vi "Initialize.vi"(8 "error in (no error)":errorcluster, 10 "Parameters in":refnum<class "Abstract Init Parameters.lvclass">, 11 "Abstract Consumer in":refnum<class "Abstract Consumer.lvclass">) -> (0 "error out":errorcluster, 3 "Abstract Consumer out":refnum<class "Abstract Consumer.lvclass">)   [LabVIEW 2017, in "Messaging.lvlib" / "Abstract Consumer.lvclass"]
uses:
  Abstract Consumer.lvclass
  Parameters/Abstract Init Parameters/Abstract Init Parameters.lvclass
  Abstract Consumer.lvclass/Abstract Consumer.ctl
  Message Queue/Abstract Message Queue/Abstract Message Queue.lvclass
  Messaging.lvlib
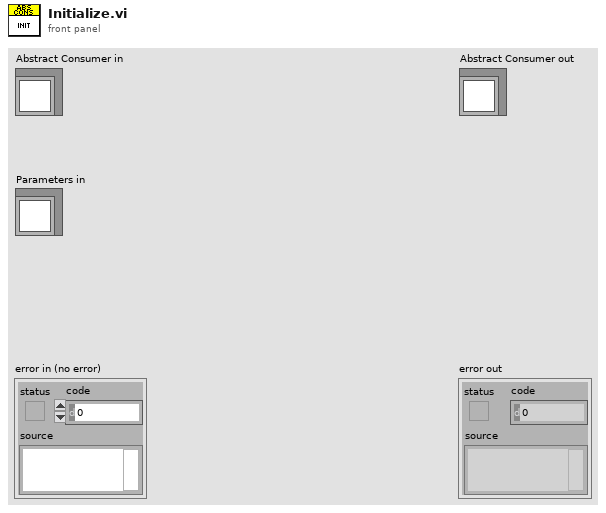
[diagram p1: front panel]
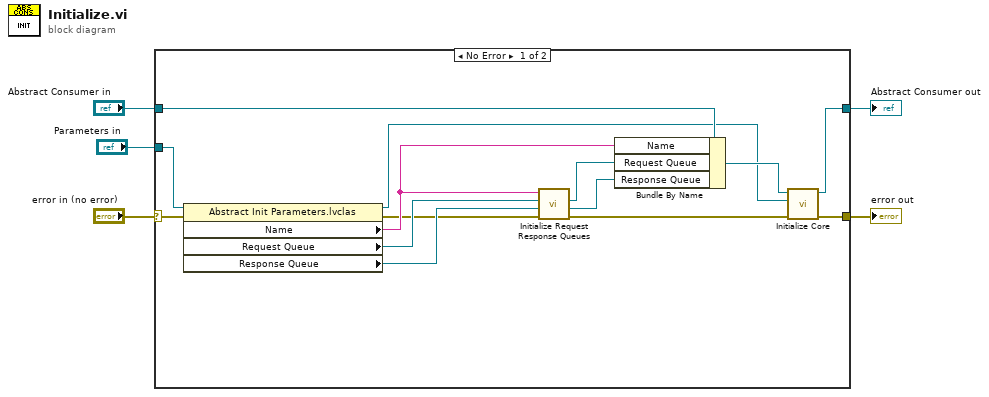
[diagram p0: block diagram]
diagram:
  n1 = case shown="No Error" "error in (no error)" {
    selector: "error in (no error)" -> [w17 w21]
    tunnel: [w9 w21] -> w4
    tunnel: [w7 w20] -> w2
    tunnel: "Abstract Consumer in" -> [w19 w20]
    tunnel: "Parameters in" -> [w18 _]
    frame No Error {
      n2 = property class="Abstract Init Parameters.lvclas"(reference=w18, error in=w17) -> (reference out=w6:refnum<class "Abstract Init Parameters.lvclass">, error out=w11:errorcluster, "Name"=w12:string, "Request Queue"=w16:refnum<class "Abstract Message Queue.lvclass">, "Response Queue"=w15:refnum<class "Abstract Message Queue.lvclass">)
      n3 = call "Initialize Request Response Queues.vi"("error in (no error)"=w11, "Response Queue in"=w15, "Request Queue in"=w16, "Name"=w12) -> ("error out"=w10:errorcluster, "Response Queue out"=w13:refnum<class "Abstract Message Queue.lvclass">, "Request Queue out"=w14:refnum<class "Abstract Message Queue.lvclass">)  [unwired: 5 in]
      n4 = Bundle By Name(cluster=w19, "Name"=w12, "Request Queue"=w14, "Response Queue"=w13) -> (w8:refnum<class "Abstract Consumer.lvclass">)
      n5 = call-dynamic "Initialize Core.vi"("error in (no error)"=w10, "Parameters"=w6, "Abstract Consumer in"=w8) -> ("error out"=w9:errorcluster, "Abstract Consumer out"=w7:refnum<class "Abstract Consumer.lvclass">)  [unwired: 7 in]
    }
    frame Error {
    }
  }
  "error out" <- w4
  "Abstract Consumer out" <- w2
